vi "Main.vi"() -> ()   [LabVIEW 2015]
uses:
  controls/Data.ctl
  support/queue state & data (Array).vi
  <vilib>/Utility/error.llb/Error Cluster From Error Code.vi
  support/queue state & data (Single).vi
  <vilib>/ErrorRing/Error Ring.xnode
  support/queue state & data.lvlib
panel:
  in  "Run Test 2":bool
  in  "Run Test 1":bool
  in  "Stop Button":bool
  # "State Machine (State & Data)"
  # "Improving string-based State Machine"
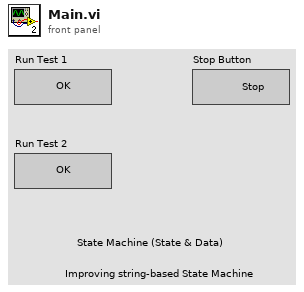
[diagram p1: front panel]
types:
  T1 = typedef "Data.ctl" = cluster{"Boolean":bool, "String":string, "Numeric":dbl, "Run Test1 Ref":refnum<vi>, "Run Test2 Ref":refnum<vi>, "Stop Butt Ref":refnum<vi>}
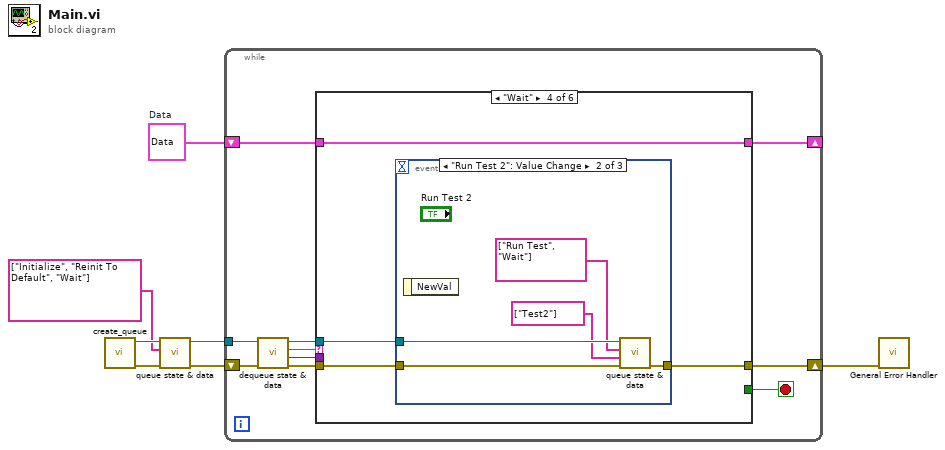
[diagram p0: block diagram]
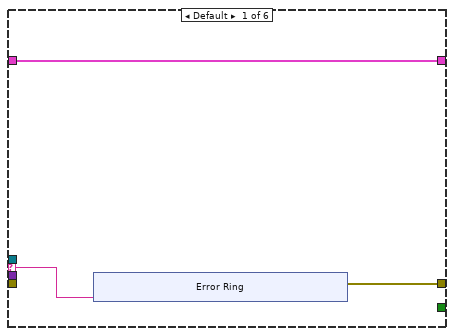
[diagram p2: hidden frame]
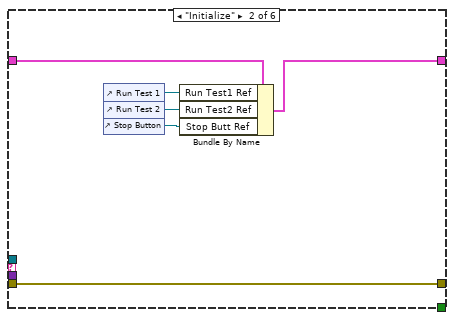
[diagram p3: hidden frame]
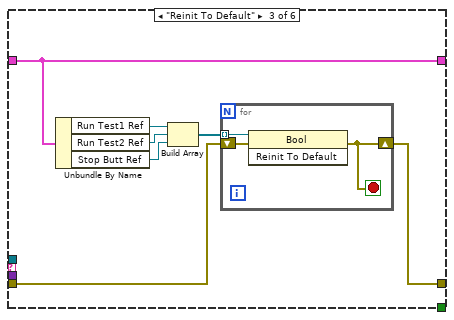
[diagram p4: hidden frame]
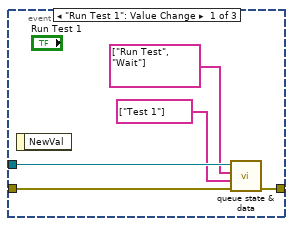
[diagram p5: hidden frame]
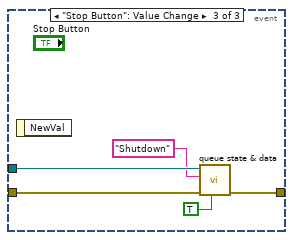
[diagram p6: hidden frame]
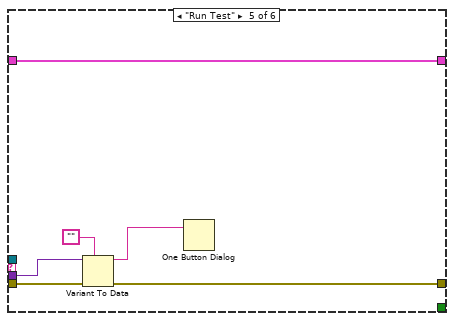
[diagram p7: hidden frame]
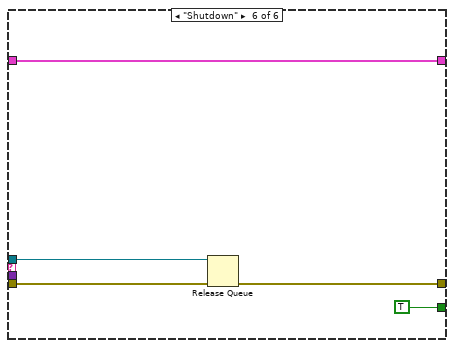
[diagram p8: hidden frame]
diagram:
  w2 = T1 {"Boolean"=FALSE, "String"="", "Numeric"=0.0, "Run Test1 Ref"=refnum, "Run Test2 Ref"=refnum, "Stop Butt Ref"=refnum}  # Data
  n1 = call "create_queue.vi"() -> ("error out"=w4:errorcluster, "queue out"=w6:refnum<queue>)  [unwired: 10 in]
  n2 = call-poly "queue state & data.vi"("error in (no error)"=w4, "State Array"=string[] ["Initialize", "Reinit To Default", "Wait"], "queue in"=w6) -> ("error out"=w5:errorcluster, "queue out"=w3:refnum<queue>)  [unwired: 7 in]
  n3 = while {
    shift-right: [w17] -> w7
    shift-left: w5 -> [w12]
    tunnel: w3 -> [w10]
    shift-right: [w8] -> _
    shift-left: w2 -> [w9]
    stop <- w16 stop-if-true
    n4 = call "dequeue state & data.vi"("error in (no error)"=w12, "queue in"=w10) -> ("error out"=w15:errorcluster, "State Data"=w13:variant, "State"=w14:string, "queue out"=w11:refnum<queue>)  [unwired: 6 in]
    n5 = case shown="\"Wait\"" w14 {
      selector: w14 -> [w19 _ _ _ _ _]
      tunnel: w15 -> [_ w28 w35 w47 w68 w72]
      tunnel: [w20 w28 w34 w46 w67 w70] -> w17
      tunnel: [_ _ _ _ _ TRUE] -> w16
      tunnel: w11 -> [_ _ _ w45 _ w71]
      tunnel: w13 -> [_ _ _ _ w66 _]
      tunnel: w9 -> [w18 w33 w40 w44 w63 w69]
      tunnel: [w18 w32 w40 w44 w63 w69] -> w8
      frame Default {
        n6 = xnode "Error Ring"("parameter 0"=w19) -> ("error out"=w20:errorcluster)
      }
      frame "Initialize" {
        n7 = control-ref of="Run Test 1"() -> (w31:refnum<vi>)
        n8 = control-ref of="Run Test 2"() -> (w30:refnum<vi>)
        n9 = control-ref of="Stop Button"() -> (w29:refnum<vi>)
        n10 = Bundle By Name(cluster=w33, "Run Test1 Ref"=w31, "Run Test2 Ref"=w30, "Stop Butt Ref"=w29) -> (w32:T1)
      }
      frame "Reinit To Default" {
        n11 = Unbundle By Name(w40) -> ("Run Test1 Ref"=w39:refnum<vi>, "Run Test2 Ref"=w38:refnum<vi>, "Stop Butt Ref"=w37:refnum<vi>)
        n12 = Build Array(w39, w38, w37) -> (w36:refnum<vi>[])
        n13 = for {
          tunnel: w36 -> [w43] mode=indexing
          shift-right: [w41] -> w34
          shift-left: w35 -> [w42]
          stop <- w41 stop-if-true
          n14 = invoke class="Bool" method="Reinit To Default"(reference=w43, error in=w42) -> (error out=w41:errorcluster)  [unwired: 1 in, 2 out]
        }
      }
      frame "Wait" {
        n15 = event shown="[1] \"Run Test 2\": Value Change" {
          selector: _ -> [_ _ _]
          dyn-events: _ -> [_ _ _]
          timeout: _ -> [_ _ _]
          tunnel: w47 -> [w52 w57 w61]
          tunnel: [w51 w56 w62] -> w46
          tunnel: w45 -> [w50 w55 w60]
          event "Run Test 1": Value Change {
            n16 = event-data() -> ()  [unwired: 1 in, 1 out]
            n17 = call-poly "queue state & data.vi"("error in (no error)"=w52, "State Data Array"=string[] ["Test 1"], "State Array"=string[] ["Run Test", "Wait"], "queue in"=w50) -> ("error out"=w51:errorcluster)  [unwired: 6 in, 1 out]
          }
          event "Run Test 2": Value Change {
            n18 = event-data() -> ()  [unwired: 1 in, 1 out]
            n19 = call-poly "queue state & data.vi"("error in (no error)"=w57, "State Data Array"=string[] ["Test2"], "State Array"=string[] ["Run Test", "Wait"], "queue in"=w55) -> ("error out"=w56:errorcluster)  [unwired: 6 in, 1 out]
          }
          event "Stop Button": Value Change {
            n20 = event-data() -> ()  [unwired: 1 in, 1 out]
            n21 = call-poly "queue state & data.vi"("Priority Message? (F)"=TRUE ("Priority? (F)"), "error in (no error)"=w61, "State"="Shutdown", "queue in"=w60) -> ("error out"=w62:errorcluster)  [unwired: 6 in, 1 out]
          }
        }
      }
      frame "Run Test" {
        n22 = Variant To Data(error in=w68, type="", Variant=w66) -> (data=w64:string, error out=w67:errorcluster)
        n23 = One Button Dialog(message=w64) -> ()  [unwired: 1 in, 1 out]
      }
      frame "Shutdown" {
        n24 = Release Queue(queue=w71, error in (no error)=w72) -> (error out=w70:errorcluster)  [unwired: 1 in, 2 out]
      }
    }
  }
  n25 = call <vilib>:"General Error Handler.vi"("error in (no error)"=w7) -> ()  [unwired: 10 in, 5 out]
